vi "Process.WriteDebugString.vi"(7 "Version":string, 8 "error in (no error)":errorcluster, 9 "State":string, 10 "severity (Informational)":i32(ring)=2 items=["Error", "Warning", "Informational"], 11 "Name":string) -> (0 "error out":errorcluster)   [LabVIEW 2025, in "xnet_can_bus_monitor_api_server_do.lvlib"]
uses:
  xnet_can_bus_monitor_api_server_do.lvlib
  <vilib>/Utility/SystemLogging/NI_SystemLogging.lvlib
panel:
  out "Debug String":string
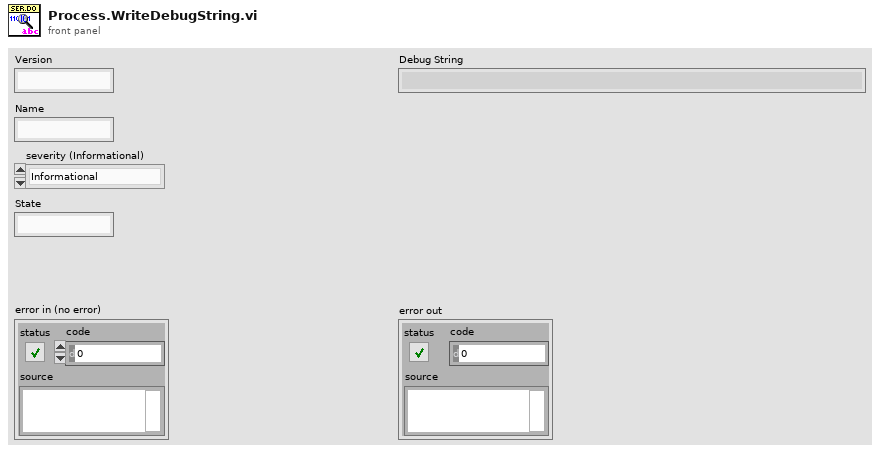
[diagram p1: front panel]
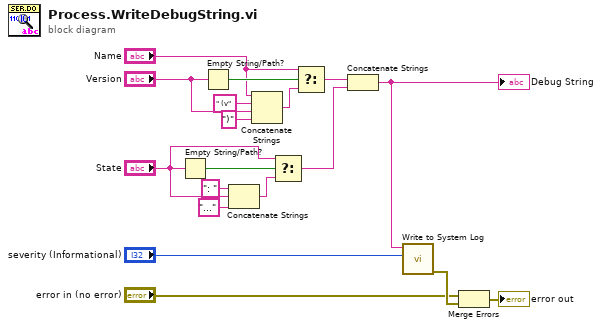
[diagram p0: block diagram]
diagram:
  n1 = Empty String/Path?(string/path="State") -> (empty?=w15:bool)
  n2 = Empty String/Path?(string/path="Version") -> (empty?=w18:bool)
  n3 = Concatenate Strings(": " ("string"), "State", "..." ("string")) -> (w13:string)
  n4 = Concatenate Strings("Name", " (v" ("string"), "Version", ")" ("string")) -> (w16:string)
  n5 = Select(t="State", s=w15, f=w13) -> (s? t:f=w12:string)
  n6 = Select(t="Name", s=w18, f=w16) -> (s? t:f=w10:string)
  n7 = Concatenate Strings(w10, w12) -> (w3:string)
  "Debug String" <- w3
  n8 = call <vilib>:"Write to System Log.vi"("severity"="severity (Informational)", "message"=w3) -> ("error out"=w7:errorcluster)  [unwired: 9 in]
  n9 = Merge Errors("error in (no error)", w7) -> (→"error out":errorcluster)
